vi "Set 2D Field (Cartesian)_brasse.vi"(2 "error in":T2, 3 "Magnitude Limit (kG)":dbl format="%.3f", 4 "Z-Axis Field (kG)":dbl format="%.3f", 6 "Z-Axis Communications Config":T1={"GPIB address"=22, "GPIB bus"=0, "connection ID"=refnum, "IP"="192.168.2.200", "Active Comm Interface"=0, "Serial Port"="", "Programmer Type"=0} {"Programmer Type" items=["Model 430", "Model 420"]; "Active Comm Interface" items=["TCP/IP (Model 430 Only)", "RS232", "IEEE488"]}, 7 "Y-Axis Field (kG)":dbl format="%.3f", 8 "Y-Axis Communications Config":T1={"GPIB address"=22, "GPIB bus"=0, "connection ID"=refnum, "IP"="192.168.2.200", "Active Comm Interface"=0, "Serial Port"="", "Programmer Type"=0} {"Programmer Type" items=["Model 430", "Model 420"]; "Active Comm Interface" items=["TCP/IP (Model 430 Only)", "RS232", "IEEE488"]}) -> (0 "error out":T2, 1 "Within Limits?":bool)   [LabVIEW 2009]
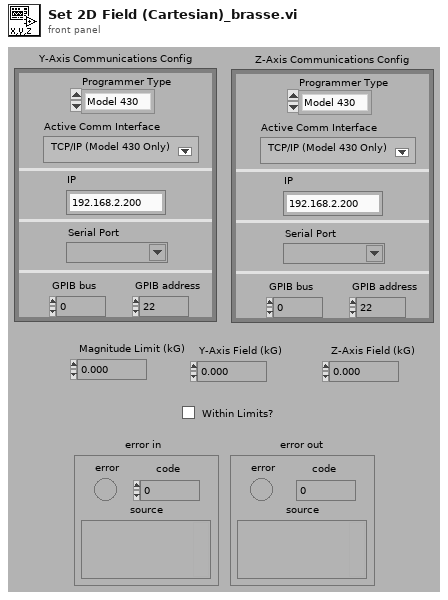
[diagram p1: front panel]
types:
  T1 = cluster{"GPIB address":i16, "GPIB bus":i16, "connection ID":refnum<k5>, "IP":string, "Active Comm Interface":u16, "Serial Port":refnum<visa-resource-name>, "Programmer Type":u16}
  T2 = cluster{"error":bool, "code":i32, "source":string}
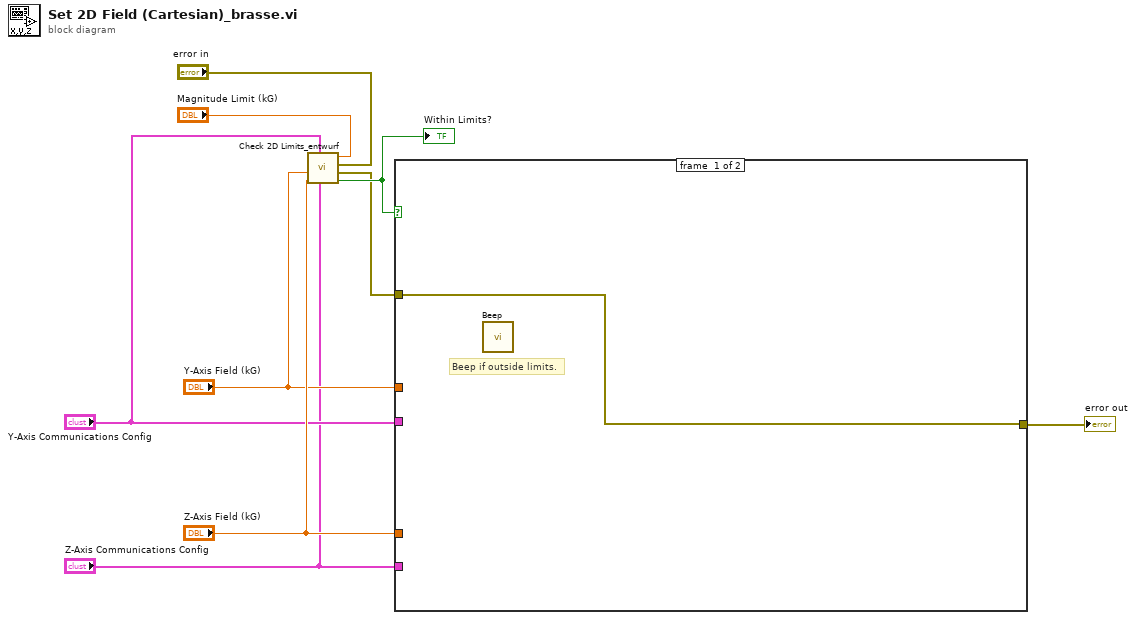
[diagram p0: block diagram]
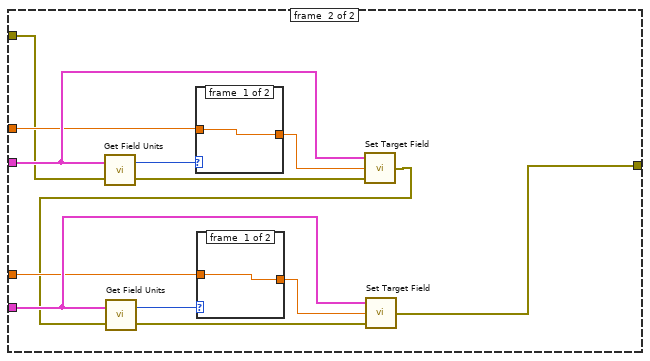
[diagram p2: hidden frame]
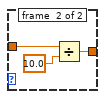
[diagram p3: hidden frame]
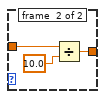
[diagram p4: hidden frame]
diagram:
  n1 = call "Check 2D Limits_entwurf.vi"("error in"="error in", "Magnitude Limit (kG)"="Magnitude Limit (kG)", "Z-Axis Communications Config"="Z-Axis Communications Config", "Y-Axis Communications Config"="Y-Axis Communications Config", "Z-Axis Field (kG)"="Z-Axis Field (kG)", "Y-Axis Field (kG)"="Y-Axis Field (kG)") -> ("Within Limits?"=w7:bool, "error out"=w4:T2)  [unwired: 2 in]
  "Within Limits?" <- w7
  n2 = case shown="False" w7 {
    tunnel: "Y-Axis Communications Config" -> [_ w17]
    tunnel: "Y-Axis Field (kG)" -> [_ w16]
    tunnel: "Z-Axis Field (kG)" -> [_ w14]
    tunnel: "Z-Axis Communications Config" -> [_ w15]
    tunnel: w4 -> [w10 w11]
    tunnel: [w10 w12] -> w8
    frame #0 {
      # "Beep if outside limits."
      n3 = call <vilib>:"Beep.vi"() -> ()  [unwired: 12 in]
    }
    frame #1 {
      n4 = call <userlib>:"Get Field Units.vi"("error in"=w11, "Communications Config"=w17) -> ("error out"=w22:T2, "Field Units"=w23:enum16{"kg", "t"})
      n5 = case shown="\"kg\", Default" w23 {
        tunnel: [w28 w30] -> w21
        tunnel: w16 -> [w28 w29]
        frame #0 {
        }
        frame #1 {
          n6 = Divide(x=w29, y=10.0) -> (x/y=w30:dbl)
        }
      }
      n7 = call <userlib>:"Set Target Field.vi"("error in"=w22, "Target Field (kG)"=w21, "Communications Config"=w17) -> ("error out"=w13:T2)
      n8 = call <userlib>:"Get Field Units.vi"("error in"=w13, "Communications Config"=w15) -> ("error out"=w19:T2, "Field Units"=w20:enum16{"kg", "t"})
      n9 = case shown="\"kg\", Default" w20 {
        tunnel: [w24 w26] -> w18
        tunnel: w14 -> [w24 w25]
        frame #0 {
        }
        frame #1 {
          n10 = Divide(x=w25, y=10.0) -> (x/y=w26:dbl)
        }
      }
      n11 = call <userlib>:"Set Target Field.vi"("error in"=w19, "Target Field (kG)"=w18, "Communications Config"=w15) -> ("error out"=w12:T2)
    }
  }
  "error out" <- w8
